vi "Digital Values.vi"(8 "error in (no error)":errorcluster, 10 "Numeric":i32=60) -> (0 "error out":errorcluster, 2 "Boolean 2":bool, 3 "Boolean":bool)   [LabVIEW 2023, in "FPGA.lvlib"]
uses:
  FPGA.lvlib
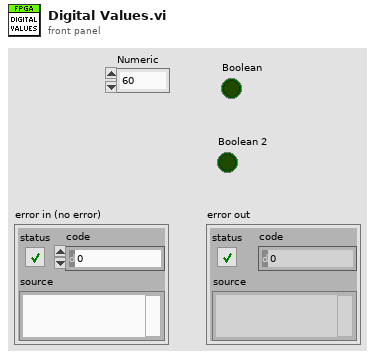
[diagram p1: front panel]
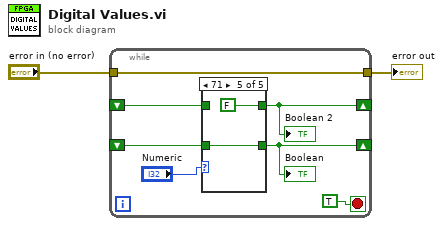
[diagram p0: block diagram]
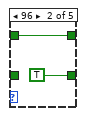
[diagram p3: hidden frame]
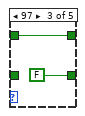
[diagram p4: hidden frame]
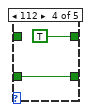
[diagram p5: hidden frame]
diagram:
  n1 = while {
    shift-right: [w7] -> _
    shift-left: _ -> [w4]
    shift-right: [w6] -> _
    shift-left: _ -> [w5]
    tunnel: "error in (no error)" -> [w3]
    tunnel: [w3] -> w1
    stop <- TRUE ("stop") stop-if-true
    n2 = case shown="71" "Numeric" {
      tunnel: [w11 TRUE ("Boolean 3") FALSE ("Boolean 3") w16 w18] -> w7
      tunnel: [w10 w12 w14 TRUE ("Boolean 2") FALSE ("Boolean 2")] -> w6
      tunnel: w5 -> [w10 w12 w14 _ _]
      tunnel: w4 -> [w11 _ _ w16 w18]
      frame 0, Default {
      }
      frame 96 {
      }
      frame 97 {
      }
      frame 112 {
      }
      frame 113 {
      }
    }
    "Boolean 2" <- w6
    "Boolean" <- w7
  }
  "error out" <- w1
